vi "Swap.vi"(8 "error in (no error)":errorcluster, 10 "Pointer b":refnum<class "Pointer.lvclass">, 11 "Pointer a":refnum<class "Pointer.lvclass">) -> (0 "error out":errorcluster, 2 "Pointer b":refnum<class "Pointer.lvclass">, 3 "Pointer a":refnum<class "Pointer.lvclass">)   [LabVIEW 2017, in "Memory Manager.lvlib" / "Pointer.lvclass"]
doc: "Swaps the address of the two provided <b>pointers</b>. This cannot be used with external pointers created via the Encapsulate method.\n\n<b>Note:</b> This VI is <b>safe</b>.\n\nSafe means that this function evaluates the size parameter of <b>pointer a</b> and <b>pointer b</b> to ensure that the memory location associated with each pointer is the same size before peforming a memory read/write. Reading/writing more data to a pointer than it has allocated can corrupt or crash LabVIEW."
uses:
  Pointer.lvclass
  Protected/Error VIs/Size Mismatch.vi
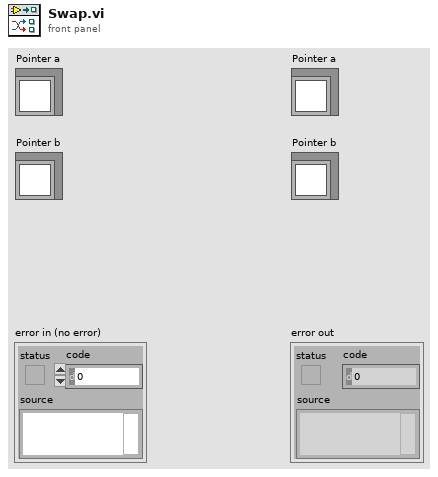
[diagram p1: front panel]
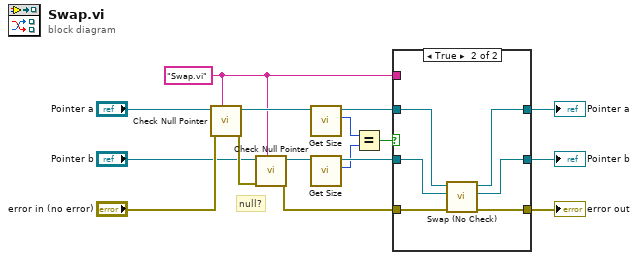
[diagram p0: block diagram]
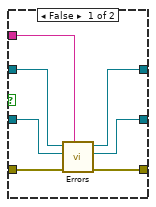
[diagram p2: hidden frame]
diagram:
  w1 = "Swap.vi" ("source vi name")
  # "null?"
  n1 = call "Check Null Pointer.vi"("source vi name"=w1, "error in (no error)"="error in (no error)", "Pointer in"="Pointer a") -> ("error out"=w5:errorcluster, "Pointer out"=w7:refnum<class "Pointer.lvclass">)  [unwired: 7 in]
  n2 = call "Check Null Pointer.vi"("source vi name"=w1, "error in (no error)"=w5, "Pointer in"="Pointer b") -> ("error out"=w3:errorcluster, "Pointer out"=w6:refnum<class "Pointer.lvclass">)  [unwired: 7 in]
  n3 = call "Get Size.vi"("Pointer in"=w7) -> ("size"=w10:u64, "Pointer out"=w15:refnum<class "Pointer.lvclass">)  [unwired: 9 in]
  n4 = call "Get Size.vi"("Pointer in"=w6) -> ("size"=w9:u64, "Pointer out"=w14:refnum<class "Pointer.lvclass">)  [unwired: 9 in]
  n5 = Equal?(x=w10, y=w9) -> (x = y?=w16:bool)
  n6 = case shown="True" w16 {
    tunnel: w15 -> [w21 w25]
    tunnel: w14 -> [w19 w29]
    tunnel: [w20 w24] -> w13
    tunnel: [w18 w28] -> w12
    tunnel: w3 -> [w23 w27]
    tunnel: [w22 w26] -> w11
    tunnel: w1 -> [w17 _]
    frame False {
      n7 = call-poly "Errors.vi"("error source vi name"=w17, "error in (no error)"=w23, "Pointer b in"=w19, "Pointer a in"=w21) -> ("error out"=w22:errorcluster, "Pointer b out"=w18:refnum<class "Pointer.lvclass">, "Pointer a out"=w20:refnum<class "Pointer.lvclass">)  [unwired: 5 in]
    }
    frame True {
      n8 = call "Swap (No Check).vi"("error in (no error)"=w27, "Pointer b"=w29, "Pointer a"=w25) -> ("error out"=w26:errorcluster, "Pointer b"=w28:refnum<class "Pointer.lvclass">, "Pointer a"=w24:refnum<class "Pointer.lvclass">)  [unwired: 6 in]
    }
  }
  "error out" <- w11
  "Pointer a" <- w13
  "Pointer b" <- w12
